vi "setAxisData.vi"() -> ()   [LabVIEW 2014]
uses:
  <vilib>/Instr/_visa.llb/VISA Configure Serial Port (Instr).vi
panel:
  out "concatenated string":string
  in  "Axis":enum16{"x", "y"}(ring)
  in  "Joystick":enum16{"left", "right"}(ring)
  in  "Set Max":bool
  in  "Set Min":bool
  out "error out":errorcluster
  in  "VISA resource name":refnum<visa-resource-name>
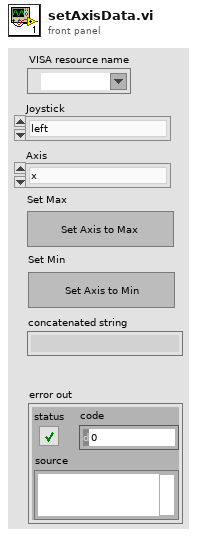
[diagram p1: front panel]
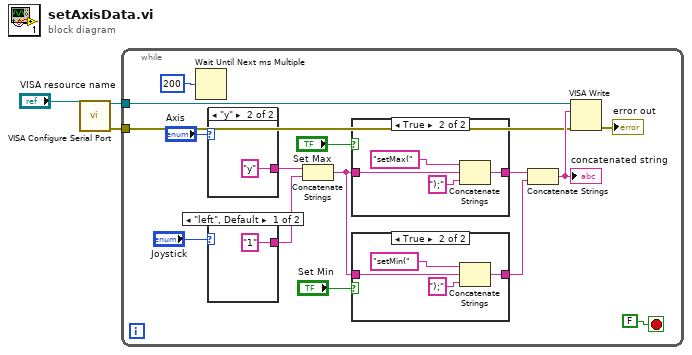
[diagram p0: block diagram]
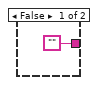
[diagram p2: hidden frame]
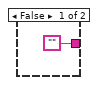
[diagram p3: hidden frame]
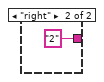
[diagram p4: hidden frame]
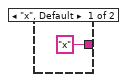
[diagram p5: hidden frame]
diagram:
  n1 = call-poly "VISA Configure Serial Port"("VISA resource name"="VISA resource name") -> ("VISA resource name out"=w2:refnum<visa-resource-name>, "error out"=w1:errorcluster)  [unwired: 13 in]
  n2 = while {
    tunnel: w2 -> [w7]
    tunnel: w1 -> [w6]
    stop <- FALSE stop-if-true
    n3 = Wait Until Next ms Multiple(millisecond multiple=u32 200) -> ()  [unwired: 1 out]
    n4 = case shown="\"y\"" "Axis" {
      tunnel: ["x" "y"] -> w16
      frame "x", Default {
      }
      frame "y" {
      }
    }
    n5 = case shown="\"left\", Default" "Joystick" {
      tunnel: ["1" "2"] -> w15
      frame "left", Default {
      }
      frame "right" {
      }
    }
    n6 = Concatenate Strings(w16, w15) -> (w13:string)
    n7 = case shown="True" "Set Max" {
      tunnel: w13 -> [_ w27]
      tunnel: ["" w25] -> w12
      frame False {
      }
      frame True {
        n8 = Concatenate Strings("setMax(", w27, ");") -> (w25:string)
      }
    }
    n9 = case shown="True" "Set Min" {
      tunnel: ["" w20] -> w11
      tunnel: w13 -> [_ w21]
      frame False {
      }
      frame True {
        n10 = Concatenate Strings("setMin(", w21, ");") -> (w20:string)
      }
    }
    n11 = Concatenate Strings(w12, w11) -> (w8:string)
    "concatenated string" <- w8
    n12 = VISA Write(VISA resource name=w7, write buffer=w8, error in (no error)=w6) -> (error out=→"error out":errorcluster)  [unwired: 2 out]
  }
